vi "New WebSocket Connection.vi"(5 "remote port":u16, 7 "remote address":string, 8 "error in (no error)":errorcluster, 9 "receive queue":refnum<queue>, 10 "send queue":refnum<queue>) -> (0 "error out":errorcluster, 3 "WebSocket Connection out":refnum<class "WebSocket Connection.lvclass">)   [LabVIEW 2019, in "WebSocket Server Toolkit.lvlib" / "WebSocket Connection.lvclass"]
doc: "<b>Description</b> (internal VI) Create a new WebSocket Connection."
uses:
  WebSocket Connection.lvclass
  types/frame_data.ctl
  WebSocket Connection.lvclass/WebSocket Connection.ctl
  WebSocket Server Toolkit.lvlib
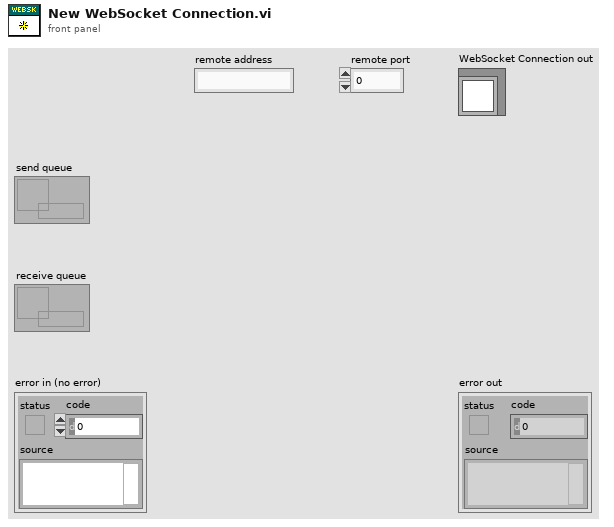
[diagram p1: front panel]
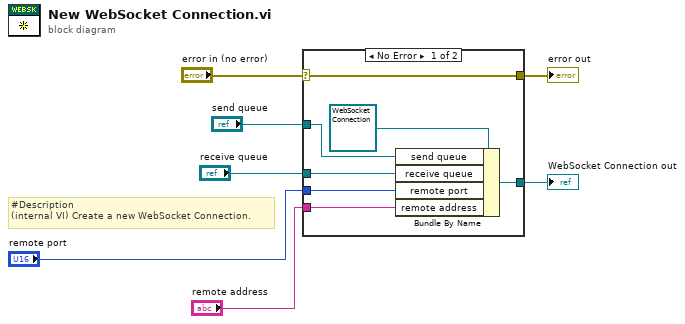
[diagram p0: block diagram]
diagram:
  # "#Description\n(internal VI) Create a new WebSocket Connection."
  n1 = case shown="No Error" "error in (no error)" {
    selector: "error in (no error)" -> [w10 w15]
    tunnel: [w10 w15] -> w6
    tunnel: [w13 _] -> w5
    tunnel: "send queue" -> [w12 _]
    tunnel: "receive queue" -> [w11 _]
    tunnel: "remote port" -> [w9 _]
    tunnel: "remote address" -> [w8 _]
    frame No Error {
      n2 = Bundle By Name(cluster=refnum<class "WebSocket Connection.lvclass"> refnum ("WebSocket Connection in"), "send queue"=w12, "receive queue"=w11, "remote port"=w9, "remote address"=w8) -> (w13:refnum<class "WebSocket Connection.lvclass">)
    }
    frame Error {
    }
  }
  "error out" <- w6
  "WebSocket Connection out" <- w5
